vi "Device VI 3.0.vi"() -> ()   [LabVIEW 2017]
uses:
  <vilib>/Math Plots/2D Math Plots/2D Compass/2D Compass XCtrl/2D Compass.xctl
  <vilib>/Math Plots/2D Math Plots/2D Compass/2D Compass Datatype/2D Compass Datatype.lvclass
  <vilib>/Utility/error.llb/DialogType.ctl
  <vilib>/DAQmx/read.llb/DAQmx Read (Digital 1D U8 1Chan NSamp).vi
  <vilib>/DAQmx/read.llb/DAQmx Read (Analog 1D Wfm NChan NSamp).vi
  <vilib>/Analysis/baseanly.llb/Mean (DBL).vi
  <vilib>/DAQmx/create/channels.llb/DAQmx Create Channel (AI-Force-Bridge-Two-Point-Linear).vi
  <vilib>/DAQmx/configure/timing.llb/DAQmx Timing (Sample Clock).vi
  <vilib>/DAQmx/configure/trigger.llb/DAQmx Start Trigger (Digital Edge).vi
  <vilib>/DAQmx/create/channels.llb/DAQmx Create Channel (AI-Voltage-Basic).vi
  <vilib>/Math Plots/2D Math Plots/2D Compass/2D Compass Datatype/Public/Plot Helper (Vector).vi
  <vilib>/DAQmx/miscellaneous.llb/DAQmx Fill In Error Info.vi
  <vilib>/Waveform/WDTFileIO.llb/Export Waveform To Spreadsheet File.vi
  <resource>/objmgr/daqmx.rc
  <vilib>/Analysis/NI_AALBase.lvlib
panel:
  in  "physical channels":tag
  in  "Digital Start Trigger Edge 2":i32(ring)=10280 caption="Edge" items=["Rising"=10280, "Falling"=10171]
  in  "Digital Start Trigger Source 2":tag="/cDAQ1Mod3/PFI0" caption="Source"
  in  "Start 2":bool
  in  "Force vs Time?":bool
  in  "Stop":bool
  out "Force Feedback":refnum<class "2D Plot Datatype.lvclass">[](xcontrol) caption="2D Compass"
  in  "scaling information":T1={"first electrical value"=0.0, "second electrical value"=1.0, "electrical units"=15897, "first physical value"=0.0, "second physical value"=7.39, "physical units"=15876} {"physical units" items=["Newtons"=15875, "Pounds"=15876, "kgf"=15877]; "electrical units" items=["Volts/Volt"=15896, "mVolts/Volt"=15897]}
  in  "Start":bool
  in  "Spreadsheet Location":path=path "C:/Users/Julio/Desktop/Device Data/Test Sheets/Test 10.csv" caption="Filename"
  in  "Maximum Force":dbl=25.0
  in  "Minimum Force":dbl=-25.0
  in  "Units (Force)":i32(ring)=15876 items=["Newtons"=15875, "Pounds"=15876, "kgf"=15877, "From Custom Scale"=10065]
  in  "Trigger Type":T2(tab)
  in  "Digital Start Trigger Edge":i32(ring)=10280 caption="Edge" items=["Rising"=10280, "Falling"=10171]
  in  "Digital Start Trigger Source":tag="/cDAQ1Mod3/PFI0" caption="Source"
  in  "Digital Pause Trigger Pause When":i32(ring)=10192 caption="Pause When" items=["High"=10192, "Low"=10214]
  in  "Digital Pause Trigger Source":tag="/Dev1/PFI0" caption="Source"
  in  "Bridge Information":T3={"Bridge Configuration"=10182, "Excitation Source"=10200, "Excitation Value"=10.0, "Nominal Resistance"=350.0} {"Excitation Source" items=["Internal"=10200, "External"=10167, "None"=10230]; "Bridge Configuration" items=["Full Bridge"=10182, "Half Bridge"=10187, "Quarter Bridge"=10270, "No Bridge"=10228]}
  in  "Physical Channel":tag="cDAQ1Mod1/ai0:1"
  in  "Sample Rate":dbl=1000.0
  in  "Samples per Loop":i32=500
  out "Force vs Time Chart":waveform(dbl)(graph)={"t0"=timestamp(3615935462.9969935 s since 1904-01-01), "dt"=0.00062, "Y"=array[500 elements], "attributes"=variant("NI_ChannelName"=variant(string "cDAQ1Mod1/ai0"), "NI_UnitDescription"=variant(string "Pounds"))} caption="Waveform Chart"
  # "Force Location"
  # "Settings"
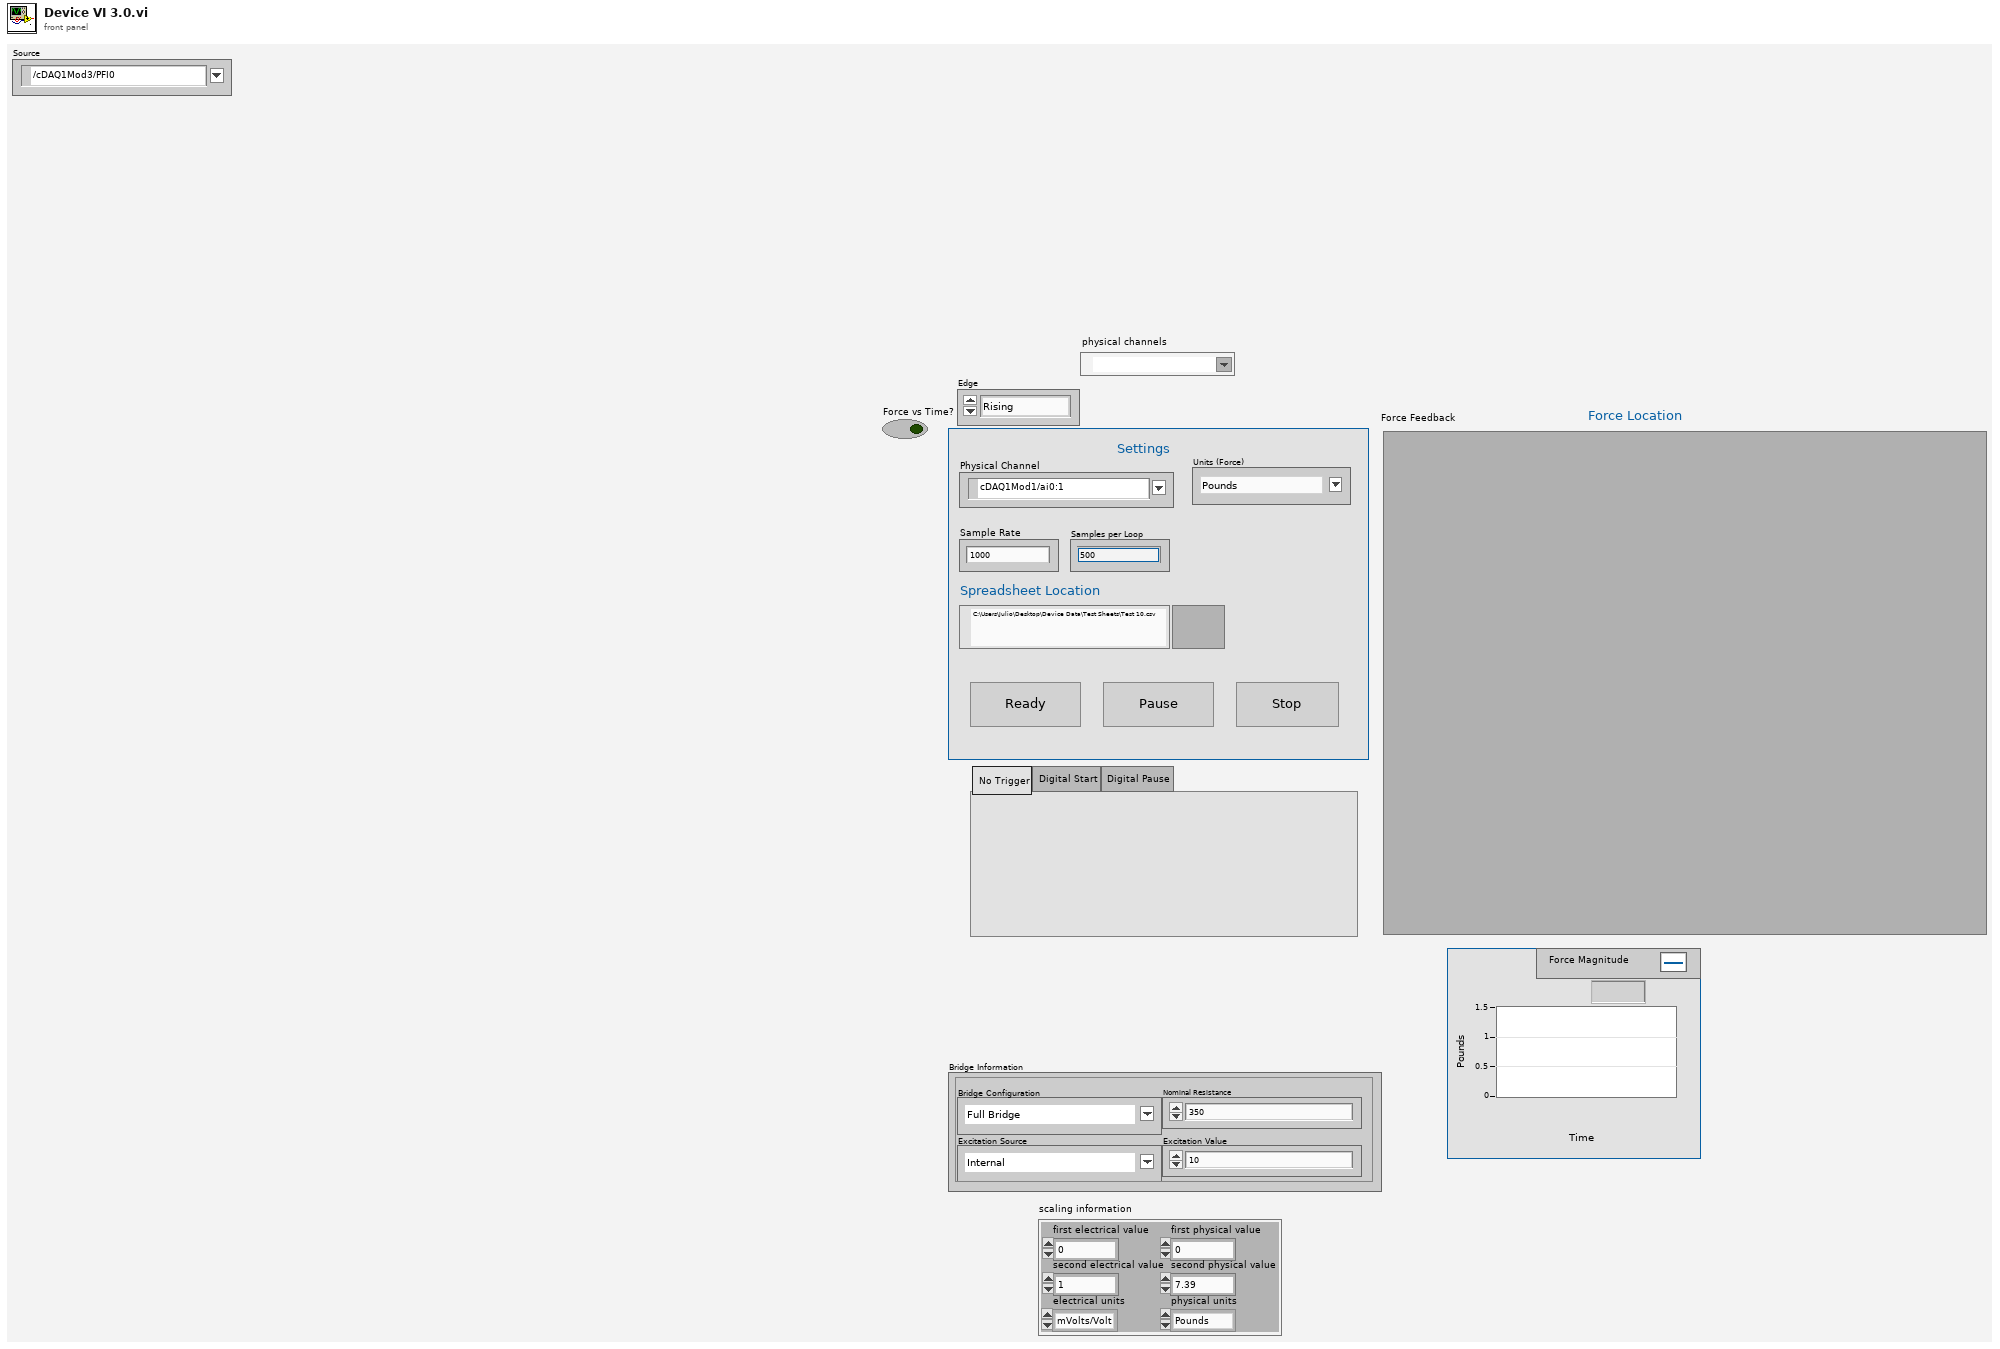
[diagram p1: front panel]
types:
  T1 = cluster{"first electrical value":dbl, "second electrical value":dbl, "electrical units":i32, "first physical value":dbl, "second physical value":dbl, "physical units":i32}
  T2 = enum32{"No Trigger", "Digital Start", "Digital Pause"}
  T3 = cluster{"Bridge Configuration":i32, "Excitation Source":i32, "Excitation Value":dbl, "Nominal Resistance":dbl}
  T4 = typedef "DialogType.ctl" = u16
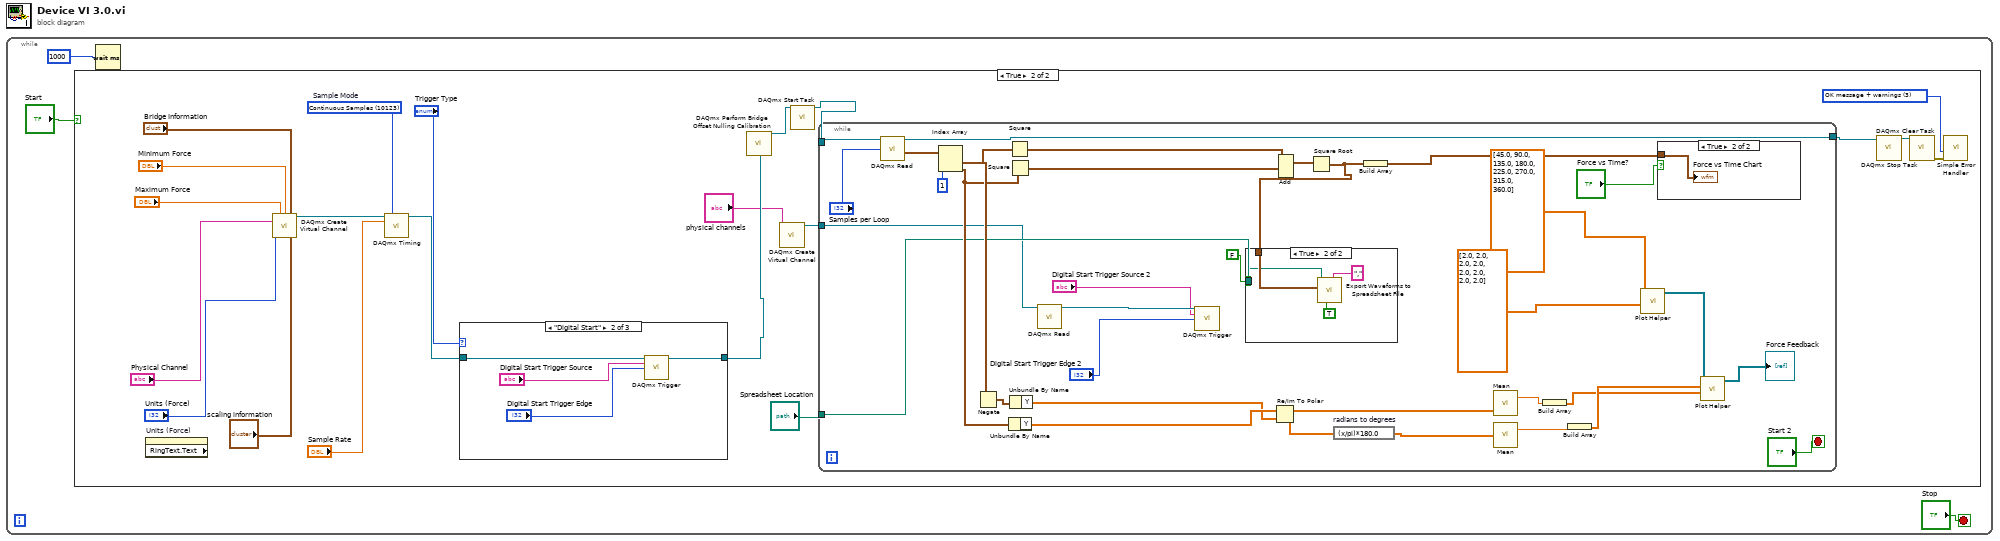
[diagram p0: block diagram]
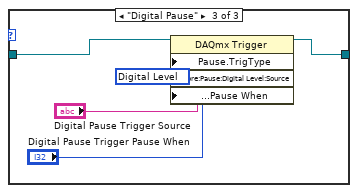
[diagram p4: hidden frame]
diagram:
  n1 = while {
    stop <- "Stop" stop-if-true
    n2 = case shown="True" "Start" {
      frame False {
      }
      frame True {
        w17 = T4 3 items=["no dialog", "OK message", "continue or stop message", "OK message + warnings", "continue/stop + warnings"] ("type of dialog (OK msg:1)")
        w24 = 10123 items=["Finite Samples"=10178, "Continuous Samples"=10123, "Hardware Timed Single Point"=12522]  # Sample Mode
        n3 = property on="Units (Force)" class="Ring (strict)" props=["RingText", "Text"]() -> ()  [unwired: 2 in, 3 out]
        n4 = call-poly <vilib>:"DAQmx Create Virtual Channel.vi"("maximum value"="Maximum Force", "minimum value"="Minimum Force", "bridge information"="Bridge Information", "physical channels"="Physical Channel", "units"="Units (Force)", "scaling information"="scaling information") -> ("task out"=w23:refnum<k21>)  [unwired: 8 in, 1 out]
        n5 = call-poly <vilib>:"DAQmx Timing.vi"("task/channels in"=w23, "sample mode"=w24, "rate"="Sample Rate") -> ("task out"=w12:refnum<k21>)  [unwired: 11 in, 1 out]
        n6 = case shown="\"Digital Start\"" "Trigger Type" {
          tunnel: w12 -> [w25 w29 w34]
          tunnel: [w25 w28 w33] -> w6
          frame "No Trigger", Default {
          }
          frame "Digital Start" {
            n7 = call-poly <vilib>:"DAQmx Trigger.vi"("task/channels in"=w29, "source"="Digital Start Trigger Source", "edge"="Digital Start Trigger Edge") -> ("task out"=w28:refnum<k21>)  [unwired: 11 in, 1 out]
          }
          frame "Digital Pause" {
            w32 = 10152 items=["Analog Level"=10101, "Analog Window"=10103, "Digital Level"=10152, "Digital Pattern"=10398, "None"=10230] ("Pause.TrigType")
            n8 = property class="DAQmx Trigger"(reference=w34, "Pause.TrigType"=w32, "More:Pause:Digital Level:Source"="Digital Pause Trigger Source", "More:Pause:Digital Level:Pause When"="Digital Pause Trigger Pause When") -> (reference out=w33:refnum<k21>)  [unwired: 1 in, 1 out]
          }
        }
        n9 = call <vilib>:"DAQmx Perform Bridge Offset Nulling Calibration.vi"("task/channels in"=w6) -> ("task out"=w9:refnum<k21>)  [unwired: 13 in, 1 out]
        n10 = call-poly <vilib>:"DAQmx Create Virtual Channel.vi"("physical channels"="physical channels") -> ("task out"=w5:refnum<k21>)  [unwired: 13 in, 1 out]
        n11 = call <vilib>:"DAQmx Start Task.vi"("task/channels in"=w9) -> ("task out"=w8:refnum<k21>)  [unwired: 13 in, 1 out]
        n12 = while {
          tunnel: w8 -> [w67]
          tunnel: "Spreadsheet Location" -> [w53]
          tunnel: [w40] -> w7
          tunnel: w5 -> [w35]
          stop <- "Start 2" stop-if-true
          n13 = call-poly <vilib>:"DAQmx Read.vi"("task/channels in"=w67, "number of samples per channel"="Samples per Loop") -> ("task out"=w40:refnum<k21>, "data"=w65:waveform(dbl)[])  [unwired: 11 in, 1 out]
          n14 = Index Array(array=w65, index #2=1 ("index")) -> (element #1=w60:waveform(dbl), element #2=w57:waveform(dbl))  [unwired: 1 in]
          n15 = Negate(x=w60) -> (-x=w58:waveform(dbl))
          n16 = Square(x=w60) -> (x^2=w62:waveform(dbl))
          n17 = Square(x=w57) -> (x^2=w63:waveform(dbl))
          n18 = Unbundle By Name(w57) -> ("Y"=w56:dbl[])
          n19 = Unbundle By Name(w58) -> ("Y"=w55:dbl[])
          n20 = call-poly <vilib>:"DAQmx Read.vi"("task/channels in"=w35) -> ("task out"=w38:refnum<k21>)  [unwired: 12 in, 2 out]
          n21 = call-poly <vilib>:"DAQmx Trigger.vi"("task/channels in"=w38, "source"="Digital Start Trigger Source 2", "edge"="Digital Start Trigger Edge 2") -> ()  [unwired: 11 in, 2 out]
          n22 = Re/Im To Polar(2:w55, 3:w56) -> (0:w54:dbl[], 1:w51:dbl[])
          n23 = Add(1:w63, 2:w62) -> (0:w64:waveform(dbl))  [unwired: 1 in, 1 out]
          n24 = Square Root(x=w64) -> (sqrt(x)=w59:waveform(dbl))
          n25 = case shown="True" FALSE {
            tunnel: w59 -> [_ w71]
            tunnel: w53 -> [_ w70]
            frame False {
            }
            frame True {
              n26 = call-poly <vilib>:"Export Waveforms to Spreadsheet File.vi"("delimiter (Tab)"=",", "append to file? (new file:F)"=TRUE, "waveform"=w71, "file path (dialog if empty)"=w70) -> ()  [unwired: 6 in, 2 out]
            }
          }
          n27 = expression code="(x/pi)*180.0" "radians to degrees"(w54) -> (w52:dbl[])
          n28 = Build Array(w59) -> ()  [unwired: 1 out]
          n29 = call-poly <vilib>:"Mean.vi"("X"=w51) -> ("mean"=w45:dbl)  [unwired: 1 out]
          n30 = call-poly <vilib>:"Mean.vi"("X"=w52) -> ("mean"=w50:dbl)  [unwired: 1 out]
          n31 = Build Array(w45) -> (w46:dbl[])
          n32 = Build Array(w50) -> (w49:dbl[])
          n33 = call-poly <vilib>:"Plot Helper.vi"("radius vector"=dbl[] [2.0, 2.0, 2.0, 2.0, 2.0, 2.0, 2.0, 2.0], "theta vector"=dbl[] [45.0, 90.0, 135.0, 180.0, 225.0, 270.0, 315.0, 360.0]) -> ("2D Plot Class Obj Array out"=w48:refnum<class "2D Plot Datatype.lvclass">[])  [unwired: 2 in, 7 out]
          n34 = case shown="True" "Force vs Time?" {
            tunnel: w59 -> [_ w72]
            frame False {
            }
            frame True {
              "Force vs Time Chart" <- w72
            }
          }
          n35 = call-poly <vilib>:"Plot Helper.vi"("radius vector"=w46, "theta vector"=w49, "2D Plot Class Obj Array in"=w48) -> ("2D Plot Class Obj Array out"=→"Force Feedback":refnum<class "2D Plot Datatype.lvclass">[])  [unwired: 1 in, 7 out]
        }
        n36 = call <vilib>:"DAQmx Stop Task.vi"("task/channels in"=w7) -> ("task out"=w18:refnum<k21>)  [unwired: 13 in, 1 out]
        n37 = call <vilib>:"DAQmx Clear Task.vi"("task in"=w18) -> ("error out"=w22:errorcluster)  [unwired: 14 in]
        n38 = call <vilib>:"Simple Error Handler.vi"("type of dialog (OK msg:1)"=w17, "error in (no error)"=w22) -> ()  [unwired: 3 in, 5 out]
      }
    }
    n39 = Wait (ms)(milliseconds to wait=u32 1000) -> ()  [unwired: 1 out]
  }
